vi "play-raster-scan-csv.vi"() -> ()   [LabVIEW 2017]
uses:
  raster-scan-params.ctl
  controls/PI-params.ctl
  controls/boolean_info.ctl
  controls/raster_input_meta_data.ctl
  <vilib>/userdefined/High Color/nirio_resource_hc.ctl
  controls/rasterMetaData.ctl
  <vilib>/Utility/file.llb/Read Delimited Spreadsheet (DBL).vi
  <vilib>/FPGAPlugInAG/cRIO-9082/niLvFpga_Open_cRIO-9082.vi
  <vilib>/rvi/interface/common/dynamic/niFpgaDynamicAddResources.vi
  <vilib>/FPGAPlugInAG/Dynamic/niLvFpga_Reset_Dynamic.vi
  <vilib>/rvi/interface/common/niFpgaWaitOnOcc.vi
  <vilib>/Utility/error.llb/Error Cluster From Error Code.vi
  <vilib>/rvi/errors/niLvFpgaAdjustHostInterfaceError.vi
  <vilib>/FPGAPlugInAG/Dynamic/niLvFpga_Run_Dynamic.vi
  fpga_interface_lib/acquire_FXP_16-5_FIFO_2.vi
  <vilib>/FPGAPlugInAG/Dynamic/niLvFpga_Close_Dynamic.vi
  <userlib>/_matio/level5/Public/Write/Append Data Element.llb/Append Data Element (Anything).vi
  <vilib>/rvi/interface/nirviOpenFPGA/nirviOpenFPGA.xnode
  FPGA Bitfiles/afmimagingcontro_FPGATargetSPARTA_raster-scanning_ejZpyk2O7fU.lvbitx
  <vilib>/rvi/interface/nirviMethod/nirviMethod.xnode
  <vilib>/rvi/interface/nirviReadWriteControl/nirviReadWriteControl.xnode
  <vilib>/rvi/interface/nirviCloseFPGA/nirviCloseFPGA.xnode
  <vilib>/FPGAPlugInAG/Dynamic/niLvFpga_ConfigureFifo_Dynamic.vi
  <vilib>/rvi/errors/niLvFpgaMergeErrorWithErrorCode.vi
  <vilib>/rvi/interface/Simulation/niFpgaSimulationCallBeginRW.vi
  fpga_interface_lib/fpga_interface.lvlib
  NiFpgaLv.dll
  <userlib>/_matio/level5.lvlib
  <vilib>/FPGAPlugInAG/Dynamic/niLvFpga_WriteFifo_Dynamic.vi
panel:
  in  "Ring 2":u16(ring) items=["x(k)", "y(k)", "deflection", "u_z"]
  in  "Alert-on-Finish":bool
  in  "do-Dz":bool
  in  "KI_derate":sgl
  in  "ze_sched_thresh":sgl
  in  "detrend":bool=TRUE
  out "InputMetaData":T1
  out "output-meta-data-path":path
  out "Tab Control":T2(tab)
  in  "input-path":path=path "Z:/afm-cs/imaging/raster/5microns/parents/raster_scan_512pix_5mic_01Hz.csv"
  in  "number-of-pixels":i32=512
  out "points_per_line":i32=250000
  out "total_num_points":i32
  in  "raise-constant (init)":sgl
  in  "raise-constant":sgl
  in  "trigger-0":bool
  in  "STOP":bool
  in  "xy-init":fxp<+/-,16,5>[](array[numeric])=[0.0, 0.0]
  in  "Ki-xy":dbl=0.015 format="%#_13g"
  out "ADC-zaxis":sgl
  out "DAC-zaxis":sgl
  in  "xy-bound":sgl=7.0
  out "output-data-path":path
  in  "note-blob":string
  in  "overwrite":bool
  in  "raster-scan-params":T3={"TsTicks"=1600, "Stop"=FALSE, "TOL"=0.3, "ramp-rate"=-0.0002, "z-u-max"=5.0, "PI-params"={"Ki"=0.01, "setpoint"=-0.3}, "Num"=[1.0237086, -2.0434425, 1.0225973, 0.0, 0.0, 0.0, 0.0, 0.0, 0.0], "TF Order"=2, "Den"=[1.0, -1.9961116, 0.998975, 0.0, 0.0, 0.0, 0.0, 0.0, 0.0]} {"ramp-rate" format="%#_5g"; "TOL" format="%#_13g"}
  in  "do_xy_CL":bool=TRUE
  out "boolean errors":T5
  in  "Z-settle-N":i16=10000
  out "Actual Depth":u32
  out "Elements Remaining":u32
  out "size(s)":i32
  out "y iter":i32
  out "nsamps 2":i32
  out "Empty Elements Remaining":u32
  out "(int) y*floor(x/y)":u64
  out "elements left 2":i32=1
  out "x >= y?":bool
  out "writing stopped":bool
  out "size(s) 2":i32
  out "case-selector-feedback":i16
  out "e(0) (threshhold init)":fxp<+/-,16,5>
  out "que timed out?":bool
  out "base y_ref (ramp)":dbl[](graph)
  out "base x_ref(triangle wave)":dbl[](graph)
  out "error":dbl[](graph)
  out "control":dbl[](graph)
  out "x":dbl[](graph)
  out "total-time":dbl
  out "Error signal (previous line) 2":dbl[](graph)
  out "Waveform Graph":dbl[](graph)
  out "Intensity Graph":dbl[][](graph)
  out "control signal (previous line)":dbl[](graph)
  # "x-axis"
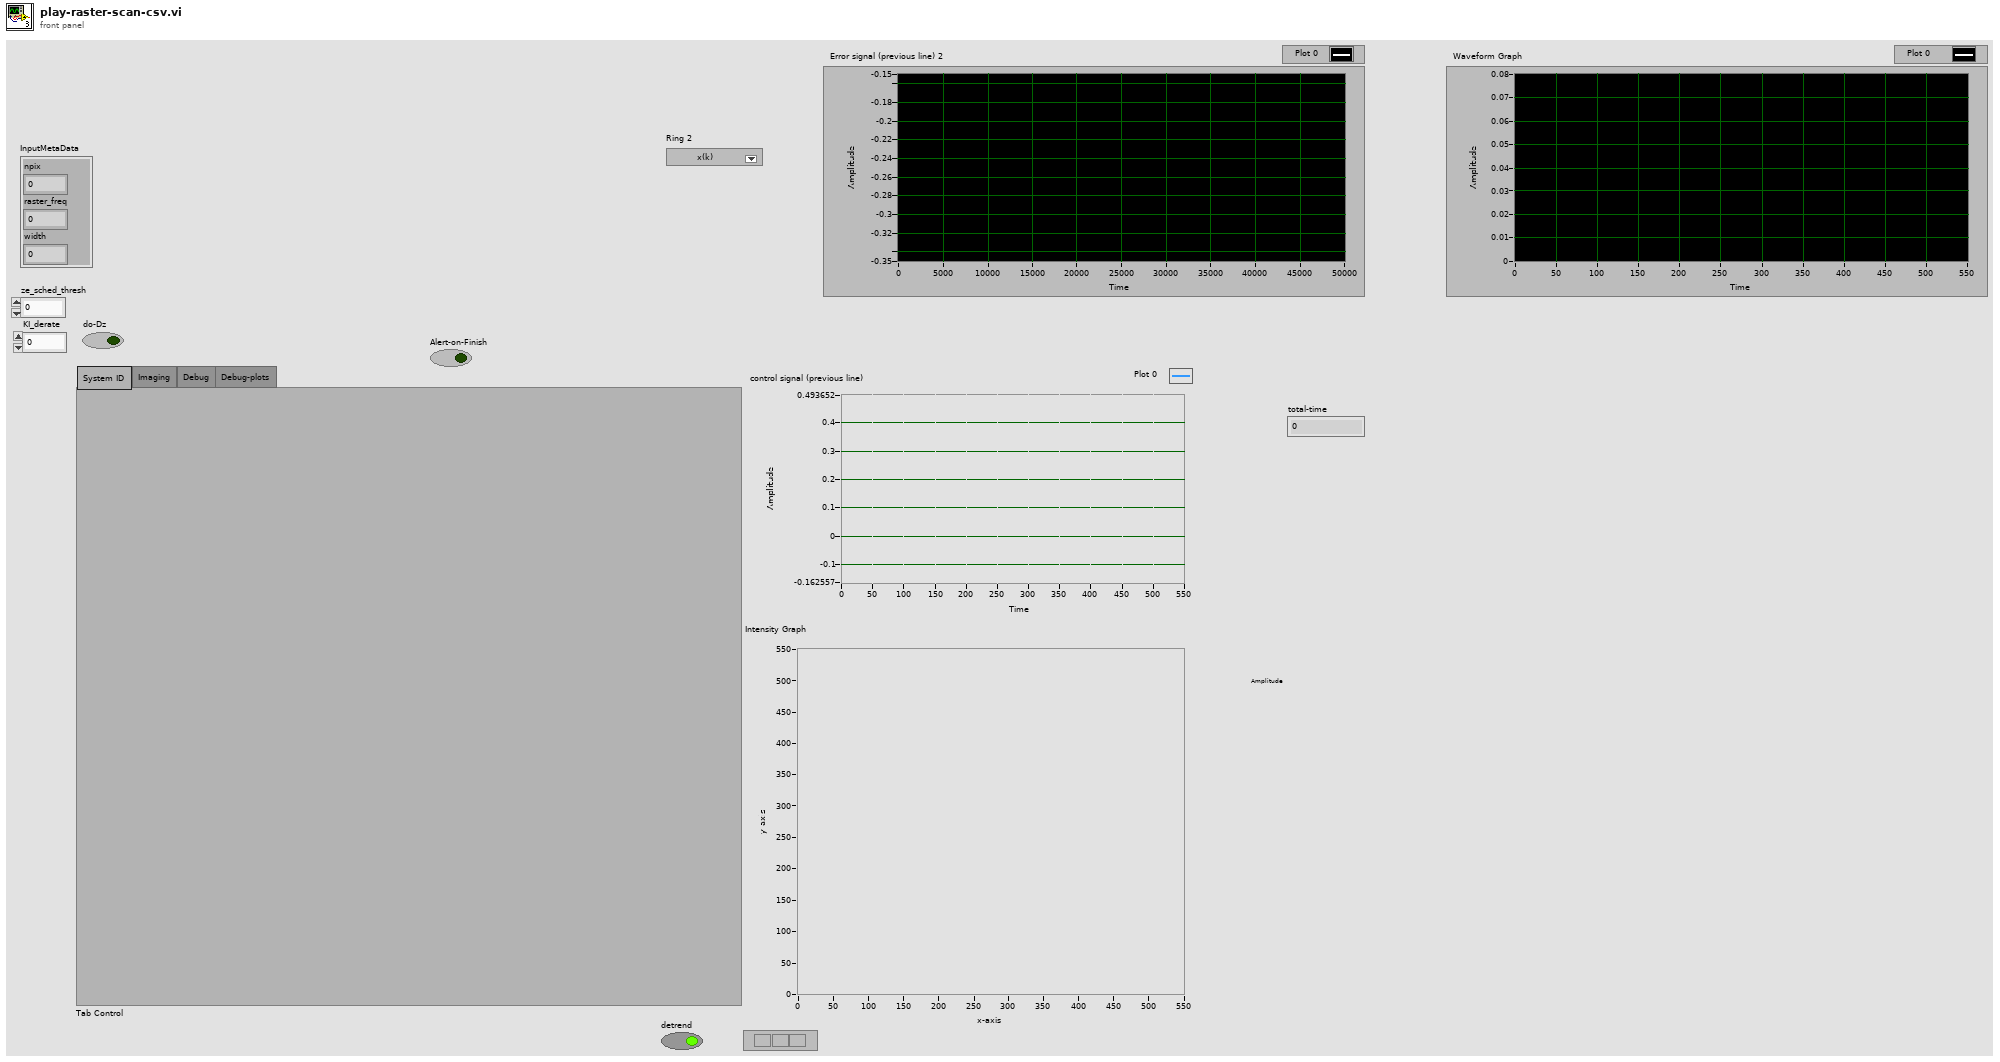
[diagram p1: front panel]
types:
  T1 = typedef "raster_input_meta_data.ctl" = cluster{"npix":dbl, "raster_freq":dbl, "width":dbl}
  T2 = enum32{"System ID", "Imaging", "Debug", "Debug-plots"}
  T3 = typedef "raster-scan-params.ctl" = cluster{"TsTicks":u32, "Stop":bool, "TOL":sgl, "ramp-rate":sgl, "z-u-max":sgl, "PI-params":T4, "Num":sgl[], "TF Order":i32, "Den":sgl[]}
  T4 = typedef "PI-params.ctl" = cluster{"Ki":sgl, "setpoint":sgl}
  T5 = typedef "boolean_info.ctl" = cluster{"unstable-z-traj":bool, "input fifo time-out":bool, "logging fifo timeout":bool, "scanning finished":bool, "unstable-x-traj":bool, "unstable-y-traj":bool, "ABORT":bool, "All Measurements Done":bool, "fpga_finished":bool}
  T6 = typedef "nirio_resource_hc.ctl" = tag
  T7 = enum16{"open", "replace", "create", "open or create", "replace or create", "replace or create with confirmation"}
  T8 = cluster{"unstable-z-traj":bool, "input fifo time-out":bool, "logging fifo timeout":bool, "scanning finished":bool, "unstable-x-traj":bool, "unstable-y-traj":bool, "ABORT":bool, "All Measurements Done":bool, "fpga_finished":bool}
  T9 = typedef "rasterMetaData.ctl" = cluster{"raster-scan-params":T3, "xy-bound":sgl, "DAC-zaxis":sgl, "ADC-zaxis":sgl, "Ki-xy":dbl, "total_num_points":i32, "points_per_line":i32, "number-of-lines":i32, "number-of-pixels":i32, "raster_meta_in":T1, "Ki-derate":sgl, "ze_sched_thresh":sgl}
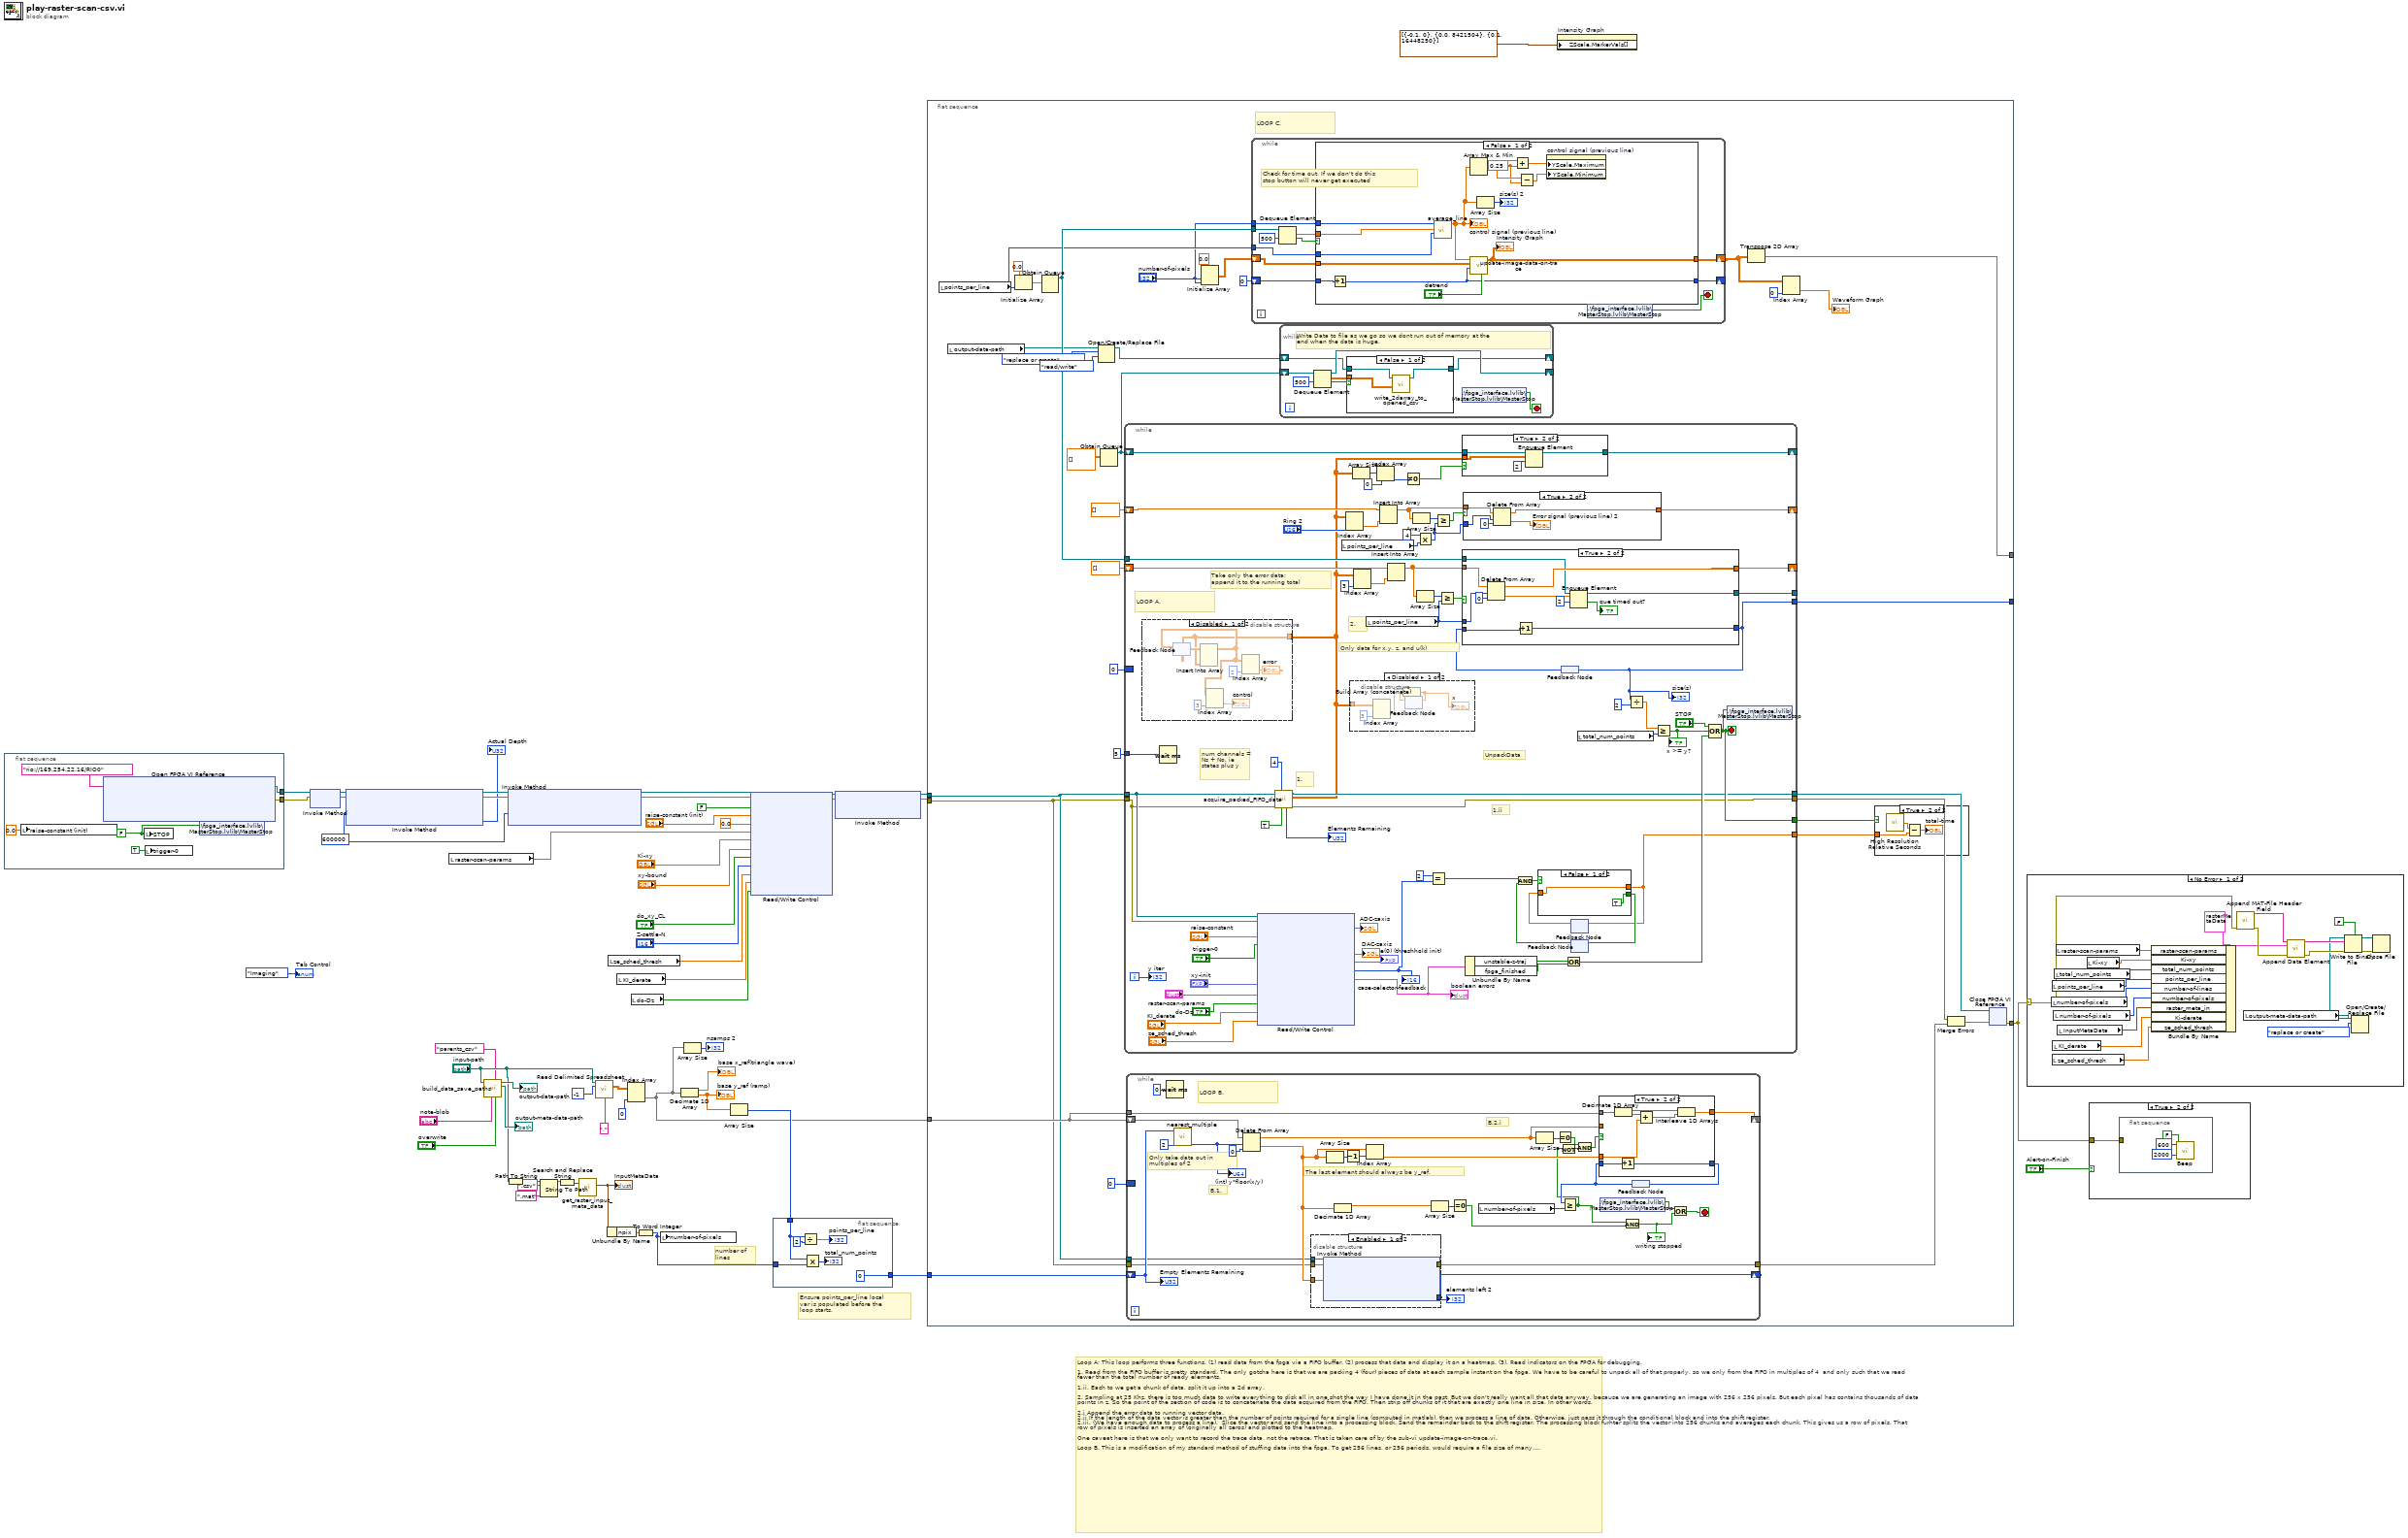
[diagram p0: block diagram]
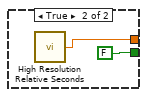
[diagram p11: hidden frame]
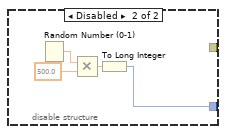
[diagram p14: hidden frame]
diagram:
  w51 = 600000
  # "number of \nlines"
  # "Loop A; This loop performs three functions. (1) read data from the fpga via a FIFO buffer. (2) process that data and display it on a heatmap. (3). Read indicators on the FPGA for debugging.\n\n1. Read from the FIFO buffer is pretty standard. The only gotcha here is that we are packing 4 (four) pieces of data at each sample instant on the fpga. We have to be careful to unpack all of that properly, so we only from the FIFO in multiples of 4  and only such that we read fewer than the total number of ready elements. \n\n1.ii. Each to we get a chunk of data, split it up into a 2d array. \n\n2. Sampling at 25 Khz, there is too much data to write everything to disk all in one shot the way I have done it in the past. But we don't really want all that data anyway, because we are generating an image with 256 x 256 pixels. But each pixel has contains thousands of data points in z. So the point of the section of code is to concatenate the data acquired from the FIFO. Then strip off chunks of it that are exactly one line in size. In other words,\n\n2.i Append the error data to running vector data.\n2.ii If the length of the data vector is greater than the number of points required for a single line (computed in matlab), then we process a line of data. Otherwise, just pass it through the conditional block and into the shift register. \n2.iii. (We have enough data to process a line).  Slice the vector and send the line into a processing block. Send the remainder back to the shift register. The processing block furhter splits the vector into 256 chunks and averages each chunk. This gives us a row of pixels. That row of pixels is inserted an array of (originally all zeros) and plotted to the heatmap.\n\nOne caveat here is that we only want to record the trace data, not the retrace. That is taken care of by the sub-vi update-image-on-trace.vi.\n\nLoop B. This is a modification of my standard method of stuffing data into the fpga. To get 256 lines, or 256 periods, would require a file size of many, many gigibtyes. SO the point here is to only use a single period of the triangle wave and corresponding ramp signal. Everytime we exauhst that data, re-cycle the same data and keep pumping it back in. The one tricky part here is that we have to be careful to shift the original ramp data up by the appropriate amount. We also have to take special care because of how the data is packed from matlab. [x(1), y(1), x(2), y(2)...].\n\nThe first iteration of the loop, we don't push any data in. All we do is get the number of empty elements.\n\nB.1 Each iteration, strip off ' empty elements ' elements from the array and send them to FIFO. \nB.2.i Is the remaining array empty?\nB.2.ii Grab the very last element. We need this"
  # "Ensure points_per_line local\nvar is populated before the\nloop starts."
  n1 = flat-sequence {
    tunnel: [w59] -> w50
    tunnel: [w58] -> w49
    frame #0 {
      w54 = FALSE
      n2 = local write "raise-constant (init)"(0.0) -> ()
      n3 = xnode "Open FPGA VI Reference"("resource name"=T6 "rio://169.254.22.16/RIO0") -> ("FPGA VI Reference Out"=w59:refnum<k20>, "error out"=w58:errorcluster)  [unwired: 1 in]
      n4 = local write "STOP"(w54) -> ()
      n5 = local write "trigger-0"(TRUE ("trigger-0")) -> ()
      n6 = shared-variable ".\\fpga_interface.lvlib\\MasterStop.lvlib\\MasterStop"(w54) -> ()  [unwired: 1 in, 1 out]
    }
  }
  n7 = xnode "Invoke Method"("FPGA VI Reference In"=w50, "error in"=w49) -> ("FPGA VI Reference Out"=w46:refnum<k20>, "error out"=w45:errorcluster)
  n8 = xnode "Invoke Method"("FPGA VI Reference In"=w46, "error in"=w45, "Requested Depth"=w51) -> ("FPGA VI Reference Out"=w47:refnum<k20>, "error out"=w48:errorcluster, "Actual Depth"=→"Actual Depth":u32)
  n9 = local read "raster-scan-params"() -> (w2:T3)
  n10 = call "build_data_save_paths.vi"("overwrite"="overwrite", "parent-subfolder-name"="parents_csv", "note-blob"="note-blob", "input-file"="input-path") -> ("output-meta-data-path"=→"output-meta-data-path":path, "output-data-path"=→"output-data-path":path)  [unwired: 4 in, 2 out]
  n11 = Path To String(path="input-path") -> (string=w18:string)
  n12 = xnode "Invoke Method"("FPGA VI Reference In"=w47, "error in"=w48, "Requested Depth"=w51) -> ("FPGA VI Reference Out"=w53:refnum<k20>, "error out"=w52:errorcluster)  [unwired: 1 out]
  n13 = Search and Replace String(input string=w18, search string=".csv", replace string=".mat" ("replace string (\"\")")) -> (result string=w15:string)  [unwired: 5 in, 3 out]
  n14 = String To Path(string=w15) -> (path=w14:path)
  n15 = call "get_raster_input_meta_data.vi"("Path"=w14) -> ("cluster"=w13:T1)  [unwired: 10 in]
  "InputMetaData" <- w13
  n16 = call-poly <vilib>:"Read Delimited Spreadsheet.vi"("file path (dialog if empty)"="input-path", "number of rows (all:-1)"=-1, "delimiter (\\t)"=",") -> ("all rows"=w32:dbl[][])  [unwired: 7 in, 5 out]
  n17 = Unbundle By Name(w13) -> ("npix"=w12:dbl)
  n18 = local read "ze_sched_thresh"() -> (w9:sgl)
  n19 = local read "KI_derate"() -> (w8:sgl)
  n20 = Index Array(array=w32, index (col)=0 ("dimension size")) -> (element=w31:dbl[])  [unwired: 1 in]
  n21 = local read "do-Dz"() -> (w10:bool)
  n22 = To Word Integer(number=w12) -> (16bit integer=w11:i16)
  n23 = local write "number-of-pixels"(w11) -> ()
  n24 = Decimate 1D Array(w31) -> (→"base x_ref(triangle wave)":dbl[], w38:dbl[])
  "base y_ref (ramp)" <- w38
  n25 = Array Size(array=w31) -> (size(s)=→"nsamps 2":i32)
  n26 = Array Size(array=w38) -> (size(s)=w36:i32)
  n27 = xnode "Read/Write Control"("FPGA VI Reference In"=w53, "error in"=w52, "trigger-0"=FALSE ("constant 2 lower"), "raise-constant"="raise-constant (init)", "u(0)"=sgl 0.0, "raster-scan-params"=w2, "Ki-xy"="Ki-xy", "xy-bound"="xy-bound", "do_xy_CL"="do_xy_CL", "Z-settle-N"="Z-settle-N", "ze_sched_thresh"=w9, "KI_derate"=w8, "do-Dz"=w10) -> ("FPGA VI Reference Out"=w28:refnum<k20>, "error out"=w27:errorcluster)
  n28 = flat-sequence {
    tunnel: [0] -> w37
    tunnel: w36 -> [w61]
    tunnel: w11 -> [w64]
    frame #0 {
      n29 = Divide(x=w61, y=2) -> (x/y=→"points_per_line":dbl)
      n30 = Multiply(x=w61, y=w64) -> (x*y=→"total_num_points":i32)
    }
  }
  n31 = xnode "Invoke Method"("FPGA VI Reference In"=w28, "error in"=w27) -> ("FPGA VI Reference Out"=w25:refnum<k20>, "error out"=w26:errorcluster)  [unwired: 1 in]
  n32 = flat-sequence {
    tunnel: [w76] -> _
    tunnel: w25 -> [w85]
    tunnel: w26 -> [w84]
    tunnel: w37 -> [w97]
    tunnel: w31 -> [w86]
    tunnel: [w70] -> _
    tunnel: [w67] -> w5
    frame #0 {
      # "LOOP C."
      n33 = local read "points_per_line"() -> (w82:i32)
      n34 = local read "output-data-path"() -> (w69:path)
      n35 = Initialize Array(0.0 ("element"), w82) -> (w91:dbl[])
      n36 = Obtain Queue(element data type=w91) -> (queue out=w88:refnum<queue>)  [unwired: 4 in, 2 out]
      n37 = Open/Create/Replace File(file path (use dialog)=w69, operation (0:open)=T7."replace or create", access (0:read/write)=enum16{"read/write", "read-only", "write-only"}."read/write") -> (refnum out=w71:refnum<file>)  [unwired: 3 in, 2 out]
      n38 = Obtain Queue(element data type=dbl[][] []) -> (queue out=w74:refnum<queue>)  [unwired: 4 in, 2 out]
      n39 = while {
        tunnel: 5 -> [w209]
        tunnel: w85 -> [w151]
        tunnel: w84 -> [w150]
        tunnel: [w148] -> w79
        tunnel: [w149] -> w80
        shift-right: [w201] -> _
        shift-left: dbl[] [] -> [w199]
        border: 0 ("disabled index (col)") -> [_]
        tunnel: w88 -> [w186]
        tunnel: [w185] -> _
        tunnel: [w152] -> w78
        tunnel: [w154] -> w77
        shift-right: [w172] -> _
        shift-left: w74 -> [w171]
        tunnel: [w170] -> w70
        shift-right: [w158] -> _
        shift-left: dbl[] [] -> [w164]
        i -> [w208]
        stop <- w152 stop-if-true
        # "2."
        # "1.ii"
        # "1."
        # "LOOP A."
        # "Take only the error data;\nappend it to the running total"
        # "num channels = Ns + No, ie states plus y"
        # "Only data for x,y, z, and u(k)"
        # "UnpackData"
        n40 = Wait (ms)(milliseconds to wait=w209) -> ()  [unwired: 1 out]
        n41 = xnode "Read/Write Control"("FPGA VI Reference In"=w151, "error in"=w150, "raise-constant"="raise-constant", "trigger-0"="trigger-0", "xy-init"="xy-init", "raster-scan-params"="raster-scan-params", "do-Dz"="do-Dz", "KI_derate"="KI_derate", "ze_sched_thresh"="ze_sched_thresh") -> ("ADC-zaxis"=→"ADC-zaxis":fxp<+/-,24,5>, "DAC-zaxis"=→"DAC-zaxis":sgl, "e(0) (threshhold init)"=→"e(0) (threshhold init)":fxp<+/-,16,5>, "current-case"=w183:i16, "boolean errors"=w169:T8)  [unwired: 2 out]
        "case-selector-feedback" <- w183
        "boolean errors" <- w169
        n42 = call-poly "acquire_packed_FIFO_data.vi"("Run once?"=TRUE, "numChannels"=u32 4 ("y"), "error in"=w150, "FPGA Interface(in)"=w151) -> ("error out"=w148:errorcluster, "2D Data Out"=w147:dbl[][], "FPGA VI Reference Out"=w149:refnum<k20>, "Elements Remaining"=→"Elements Remaining":u32)  [unwired: 3 in, 1 out]
        n43 = disable-structure shown="Disabled" {
          disable-tunnel: w147 -> [w221 _]
          frame Disabled {
            n44 = feedback #1(w221) -> (w227:dbl[][])
            n45 = Insert Into Array(array=w227, new element=w221) -> (w222:dbl[][])  [unwired: 2 in]
            n46 = feedback-in #1(w222) -> ()
            n47 = Index Array(array=w222, index (col)=3 ("disabled index (col)")) -> (element=→"control":dbl[])  [unwired: 1 in]
            n48 = Index Array(array=w222, index (col)=2 ("disabled index (col)")) -> (element=→"error":dbl[])  [unwired: 1 in]
          }
          frame Enabled {
          }
        }
        n49 = local read "points_per_line"() -> (w162:i32)
        n50 = Index Array(array=w147, index (col)="Ring 2") -> (element=w165:dbl[])  [unwired: 1 in]
        n51 = disable-structure shown="Disabled" {
          disable-tunnel: w147 -> [w219 _]
          frame Disabled {
            n52 = Index Array(array=w219, index (col)=3 ("disabled index (col)")) -> (element=w218:dbl[])  [unwired: 1 in]
            n53 = feedback #2() -> (w217:dbl[])  [unwired: 1 in]
            n54 = Build Array (concatenate)(w218, w217) -> (w216:dbl[])
            "x" <- w216
            n55 = feedback-in #2(w216) -> ()
          }
          frame Enabled {
          }
        }
        n56 = Array Size(array=w147) -> (size(s)=w176:i32[])
        n57 = Index Array(array=w147, index (col)=3 ("disabled index (col)")) -> (element=w198:dbl[])  [unwired: 1 in]
        n58 = local read "points_per_line"() -> (w191:i32)
        n59 = Index Array(array=w176, index=0) -> (element=w174:i32)
        n60 = Insert Into Array(array=w164, new element=w165) -> (w159:dbl[])  [unwired: 1 in]
        n61 = Insert Into Array(array=w199, new element=w198) -> (w177:dbl[])  [unwired: 1 in]
        n62 = Not Equal To 0?(x=w174) -> (x != 0?=w173:bool)
        n63 = Array Size(array=w159) -> (size(s)=w163:i32)
        n64 = Array Size(array=w177) -> (size(s)=w200:i32)
        n65 = Multiply(x=4, y=w162) -> (x*y=w157:i32)
        n66 = Equal?(x=i16 2, y=w183) -> (x = y?=w181:bool)
        n67 = Greater Or Equal?(x=w163, y=w157) -> (x >= y?=w160:bool)
        n68 = Greater Or Equal?(x=w200, y=w191) -> (x >= y?=w197:bool)
        n69 = case shown="True" w173 {
          tunnel: w171 -> [w228 w232]
          tunnel: w147 -> [_ w230]
          tunnel: [w228 w229] -> w172
          frame False {
          }
          frame True {
            n70 = Enqueue Element(queue=w232, element=w230, timeout in ms (-1)=2) -> (queue out=w229:refnum<queue>)  [unwired: 1 in, 2 out]
          }
        }
        n71 = case shown="True" w160 {
          tunnel: w159 -> [w210 w215]
          tunnel: [w210 w212] -> w158
          tunnel: w157 -> [_ w213]
          frame False {
          }
          frame True {
            n72 = Delete From Array(array=w215, length=w213, index=0) -> (deleted portion=→"Error signal (previous line) 2":dbl[], array with subset deleted=w212:dbl[])
          }
        }
        n73 = Unbundle By Name(w169) -> ("unstable-z-traj"=w188:bool, "fpga_finished"=w187:bool)
        n74 = feedback #3() -> (w196:i32)
        n75 = case shown="True" w197 {
          tunnel: [w239 w248] -> w201
          tunnel: w177 -> [w239 w250]
          tunnel: w196 -> [w238 w247]
          tunnel: [w238 w246] -> w170
          tunnel: w191 -> [_ w245]
          tunnel: w186 -> [w237 w243]
          tunnel: [w237 w242] -> w185
          frame False {
          }
          frame True {
            n76 = Delete From Array(array=w250, length=w245, index=0) -> (deleted portion=w244:dbl[], array with subset deleted=w248:dbl[])
            n77 = Increment(x=w247) -> (x+1=w246:i32)
            n78 = Enqueue Element(queue=w243, element=w244, timeout in ms (-1)=2) -> (queue out=w242:refnum<queue>, timed out?=→"que timed out?":bool)  [unwired: 1 in, 1 out]
          }
        }
        "size(s)" <- w170
        n79 = feedback-in #3(w170) -> ()
        n80 = Or(x=w188, y=w187) -> (x .or. y?=w192:bool)
        n81 = feedback #4() -> (w153:dbl)  [unwired: 1 in]
        n82 = feedback #5() -> (w179:bool)  [unwired: 1 in]
        n83 = And(x=w181, y=w179) -> (x .and. y?=w182:bool)
        n84 = case shown="False" w182 {
          tunnel: [TRUE FALSE] -> w180
          tunnel: [w233 w235] -> w154
          tunnel: w153 -> [w233 _]
          frame False {
          }
          frame True {
            n85 = call <vilib>:"High Resolution Relative Seconds.vi"() -> ("relative seconds"=w235:dbl)
          }
        }
        n86 = feedback-in #4(w154) -> ()
        n87 = feedback-in #5(w180) -> ()
        n88 = local read "total_num_points"() -> (w195:i32)
        n89 = Divide(x=w170, y=2) -> (x/y=w190:dbl)
        n90 = Greater Or Equal?(x=w190, y=w195) -> (x >= y?=w193:bool)
        "x >= y?" <- w193
        n91 = Compound Arithmetic op=OR("STOP", w193, w192) -> (w152:bool)
        n92 = shared-variable ".\\fpga_interface.lvlib\\MasterStop.lvlib\\MasterStop"(w152) -> ()  [unwired: 1 in, 1 out]
        "y iter" <- w208
      }
      n93 = while {
        shift-right: [w280] -> _
        shift-left: w97 -> [w276]
        shift-right: [w269] -> _
        shift-left: w86 -> [w281]
        tunnel: w86 -> [w267]
        tunnel: [w273] -> w98
        tunnel: w85 -> [w265]
        tunnel: w84 -> [w264]
        border: 0 ("Timeout (ms)") -> [_]
        stop <- w277 stop-if-true
        # "B.2.i"
        # "B.1."
        # "LOOP B."
        # "Only take data out in \nmultiples of 2"
        # "The last element should always be y_ref."
        n94 = Wait (ms)(milliseconds to wait=0) -> ()  [unwired: 1 out]
        n95 = call "nearest_multiple.vi"("numChan"=u32 2 ("Empty Elements Remaining"), "N"=w276) -> ("(int) y*floor(x/y)"=w275:u64)  [unwired: 9 in]
        "(int) y*floor(x/y)" <- w275
        n96 = Delete From Array(array=w281, length=w275, index=0) -> (deleted portion=w270:dbl[], array with subset deleted=w268:dbl[])
        n97 = disable-structure shown="Enabled" {
          disable-tunnel: [w296 w297] -> w280
          disable-tunnel: w270 -> [w295 _]
          disable-tunnel: [w294 _] -> w273
          disable-tunnel: w265 -> [w293 _]
          disable-tunnel: w264 -> [w292 _]
          frame Enabled {
            n98 = xnode "Invoke Method"("FPGA VI Reference In"=w293, "error in"=w292, "Data"=w295) -> ("error out"=w294:errorcluster, "Empty Elements Remaining"=w296:u32)  [unwired: 1 in, 1 out]
          }
          frame Disabled {
            n99 = Random Number (0-1)() -> (number: 0 to 1=w300:dbl)
            n100 = Multiply(x=w300, y=500.0) -> (x*y=w298:dbl)
            n101 = To Long Integer(number=w298) -> (32bit integer=w297:i32)
          }
        }
        "elements left 2" <- w280
        n102 = Array Size(array=w270) -> (size(s)=w271:i32)
        n103 = Decimate 1D Array(w270) -> (w256:dbl[])  [unwired: 1 out]
        n104 = Decrement(x=w271) -> (x-1=w272:i32)
        n105 = Index Array(array=w270, index=w272) -> (element=w266:dbl)
        n106 = Array Size(array=w256) -> (size(s)=w258:i32)
        n107 = Equal To 0?(x=w258) -> (x = 0?=w257:bool)
        n108 = local read "number-of-pixels"() -> (w262:i32)
        n109 = Array Size(array=w268) -> (size(s)=w278:i32)
        n110 = Equal To 0?(x=w278) -> (x = 0?=w255:bool)
        n111 = shared-variable ".\\fpga_interface.lvlib\\MasterStop.lvlib\\MasterStop"() -> (w251:bool)  [unwired: 1 in, 1 out]
        n112 = feedback #6() -> (w260:i32)
        n113 = Greater Or Equal?(x=w260, y=w262) -> (x >= y?=w253:bool)
        n114 = Not(x=w253) -> (.not. x?=w254:bool)
        n115 = And(x=w255, y=w254) -> (x .and. y?=w252:bool)
        n116 = case shown="True" w252 {
          tunnel: [w283 w286] -> w269
          tunnel: w268 -> [w283 _]
          tunnel: w267 -> [_ w291]
          tunnel: w266 -> [_ w289]
          tunnel: [w282 w285] -> w261
          tunnel: w260 -> [w282 w284]
          frame False {
          }
          frame True {
            n117 = Decimate 1D Array(w291) -> (w288:dbl[], w290:dbl[])
            n118 = Increment(x=w284) -> (x+1=w285:i32)
            n119 = Add(x=w290, y=w289) -> (x+y=w287:dbl[])
            n120 = Interleave 1D Arrays(w288, w287) -> (w286:dbl[])
          }
        }
        n121 = And(x=w253, y=w257) -> (x .and. y?=w259:bool)
        "writing stopped" <- w259
        n122 = feedback-in #6(w261) -> ()
        n123 = Or(x=w251, y=w259) -> (x .or. y?=w277:bool)
        "Empty Elements Remaining" <- w276
      }
      n124 = Initialize Array(0.0 ("element"), "number-of-pixels", "number-of-pixels") -> (w90:dbl[][])
      n125 = while {
        shift-right: [w126] -> w87
        shift-left: w90 -> [w125]
        shift-right: [w123] -> _
        shift-left: 0 ("disabled index (col)") -> [w124]
        tunnel: w82 -> [w122]
        tunnel: w88 -> [w121]
        tunnel: "number-of-pixels" -> [w117]
        stop <- w116 stop-if-true
        # "Check for time out. If we don't do this\nstop button will never get executed"
        n126 = Dequeue Element(queue=w121, timeout in ms (-1)=500) -> (element=w120:dbl[], timed out?=w118:bool)  [unwired: 1 in, 2 out]
        n127 = case shown="False" w118 {
          tunnel: [w141 w142] -> w126
          tunnel: w125 -> [w140 w142]
          tunnel: w124 -> [w139 w143]
          tunnel: [w128 w143] -> w123
          tunnel: w122 -> [w138 _]
          tunnel: w120 -> [w137 _]
          tunnel: w117 -> [w135 _]
          frame False {
            w129 = 0.25
            n128 = Increment(x=w139) -> (x+1=w128:i32)
            n129 = call "average_line.vi"("data-pts-per-line"=w138, "raw-data-row"=w137, "number-of-pixels"=w135) -> ("avg-data-row"=w127:dbl[])  [unwired: 8 in]
            "control signal (previous line)" <- w127
            n130 = Array Max & Min(array=w127) -> (max value=w133:dbl, min value=w130:dbl)  [unwired: 2 out]
            n131 = call "update-image-data-on-trace.vi"("detrend"="detrend", "iterator"=w128, "master-image-data-n"=w140, "avg-data-row"=w127) -> ("master-image-data-out"=w141:dbl[][])  [unwired: 7 in]
            "Intensity Graph" <- w141
            n132 = Array Size(array=w127) -> (size(s)=→"size(s) 2":i32)
            n133 = Add(x=w133, y=w129) -> (x+y=w132:dbl)
            n134 = Subtract(x=w130, y=w129) -> (x-y=w131:dbl)
            n135 = property on="control signal (previous line)" class="WFGraph (strict)"("YScale.Maximum"=w132, "YScale.Minimum"=w131) -> ()  [unwired: 2 in, 2 out]
          }
          frame True {
          }
        }
        n136 = shared-variable ".\\fpga_interface.lvlib\\MasterStop.lvlib\\MasterStop"() -> (w116:bool)  [unwired: 1 in, 1 out]
      }
      n137 = while {
        shift-right: [w104] -> _
        shift-left: w74 -> [w105]
        shift-right: [w102] -> _
        shift-left: w71 -> [w103]
        stop <- w101 stop-if-true
        # "Write Data to file as we go so we dont run out of memory at the \nend when the data is huge."
        n138 = Dequeue Element(queue=w105, timeout in ms (-1)=500) -> (queue out=w104:refnum<queue>, element=w106:dbl[][], timed out?=w107:bool)  [unwired: 1 in, 1 out]
        n139 = case shown="False" w107 {
          tunnel: w106 -> [w109 _]
          tunnel: w103 -> [w111 w112]
          tunnel: [w110 w112] -> w102
          frame False {
            n140 = call "write_2darray_to_opened_csv.vi"("Data_in"=w109, "file_ref_in"=w111) -> ("file_ref_out"=w110:refnum<file>)  [unwired: 8 in, 1 out]
          }
          frame True {
          }
        }
        n141 = shared-variable ".\\fpga_interface.lvlib\\MasterStop.lvlib\\MasterStop"() -> (w101:bool)  [unwired: 1 in, 1 out]
      }
      n142 = Transpose 2D Array(2D array=w87) -> (transposed array=w76:dbl[][])
      n143 = Index Array(array=w87, index (col)=0 ("disabled index (col)")) -> (element=→"Waveform Graph":dbl[])  [unwired: 1 in]
      n144 = case shown="True" w78 {
        tunnel: w77 -> [_ w115]
        frame False {
        }
        frame True {
          n145 = call <vilib>:"High Resolution Relative Seconds.vi"() -> ("relative seconds"=w114:dbl)
          n146 = Subtract(x=w114, y=w115) -> (x-y=→"total-time":dbl)
        }
      }
      n147 = Merge Errors(w79, w98) -> (w68:errorcluster)
      n148 = xnode "Close FPGA VI Reference"("FPGA VI Reference In"=w80, "error in"=w68) -> ("error out"=w67:errorcluster)
    }
  }
  n149 = property on="Intensity Graph" class="IntGraph (strict)"("ZScale.MarkerVals[]"=cluster{dbl, u32}[] [{-0.1, 0}, {0.0, 8421504}, {0.1, 16448250}] ("Z Scale.Marker Values[]")) -> ()  [unwired: 2 in, 2 out]
  n150 = case shown="No Error" w5 {
    selector: w5 -> [w311 _]
    frame No Error {
      n151 = local read "number-of-pixels"() -> (w305:i32)
      n152 = local read "points_per_line"() -> (w306:i32)
      n153 = local read "ze_sched_thresh"() -> (w301:sgl)
      n154 = local read "KI_derate"() -> (w302:sgl)
      n155 = local read "number-of-pixels"() -> (w304:i32)
      n156 = local read "total_num_points"() -> (w307:i32)
      n157 = local read "raster-scan-params"() -> (w309:T3)
      n158 = local read "InputMetaData"() -> (w303:T1)
      n159 = local read "Ki-xy"() -> (w308:dbl)
      n160 = Bundle By Name(cluster=T9 {"raster-scan-params"={"TsTicks"=1600, "Stop"=TRUE, "TOL"=0.3, "ramp-rate"=-5e-05, "z-u-max"=5.0, "PI-params"={"Ki"=0.01, "setpoint"=0.0}, "Num"=[1.0, 0.0, 0.0, 0.0, 0.0, 0.0, 0.0, 0.0, 0.0], "TF Order"=3, "Den"=[1.0, 0.0, 0.0, 0.0, 0.0, 0.0, 0.0, 0.0, 0.0]}, "xy-bound"=7.0, "DAC-zaxis"=0.0, "ADC-zaxis"=0.0, "Ki-xy"=0.01, "total_num_points"=0, "points_per_line"=250000, "number-of-lines"=256, "number-of-pixels"=256, "raster_meta_in"={"npix"=0.0, "raster_freq"=0.0, "width"=0.0}, "Ki-derate"=0.01, "ze_sched_thresh"=0.0} ("Cluster"), "raster-scan-params"=w309, "Ki-xy"=w308, "total_num_points"=w307, "points_per_line"=w306, "number-of-lines"=w305, "number-of-pixels"=w304, "raster_meta_in"=w303, "Ki-derate"=w302, "ze_sched_thresh"=w301) -> (w310:T9)
      n161 = call <userlib>:"Append MAT-File Header Field.vi"("error"=w311) -> ("result string"=w322:string, "error out"=w316:errorcluster)  [unwired: 13 in]
      n162 = local read "output-meta-data-path"() -> (w313:path)
      n163 = call-poly <userlib>:"Append Data Element.vi"("initial string"=w322, "data"=w310, "error in (no error)"=w316) -> ("result string"=w320:string, "error out"=w321:errorcluster)  [unwired: 11 in]
      n164 = Open/Create/Replace File(file path (use dialog)=w313, operation (0:open)=T7."replace or create") -> (refnum out=w315:refnum<file>)  [unwired: 4 in, 2 out]
      n165 = Write to Binary File(file (use dialog)=w315, data=w320, error in=w321, 5:FALSE ("prepend array or string size? (T)")) -> (refnum out=w317:refnum<file>, error out=w318:errorcluster)  [unwired: 2 in, 1 out]
      n166 = Close File(refnum=w317, error in=w318) -> ()  [unwired: 2 out]
    }
    frame Error {
    }
  }
  n167 = case shown="True" "Alert-on-Finish" {
    tunnel: w5 -> [_ w323]
    frame False {
    }
    frame True {
      n168 = flat-sequence {
        tunnel: w323 -> [_]
        frame #0 {
          n169 = call <vilib>:"Beep.vi"("use system alert? (T)"=FALSE, "duration (msec)"=u32 2000, "frequency (Hz)"=u32 600) -> ()  [unwired: 9 in]
        }
      }
    }
  }
  "Tab Control" <- enum32{"System ID", "Imaging", "Debug"}."Imaging" ("Tab Control")
